vi "LVIS_VerifyTests.vi"(8 "Error In":errorcluster) -> (0 "Error Out":errorcluster)   [LabVIEW 2015]
doc: "Organizes the test and measurement data and verifies it is valid."
uses:
  Globals/LVIS_IsGlobal.vi
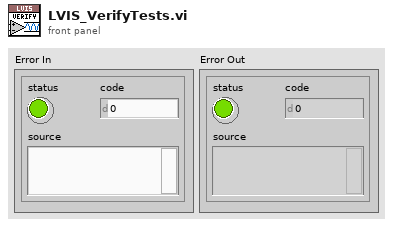
[diagram p1: front panel]
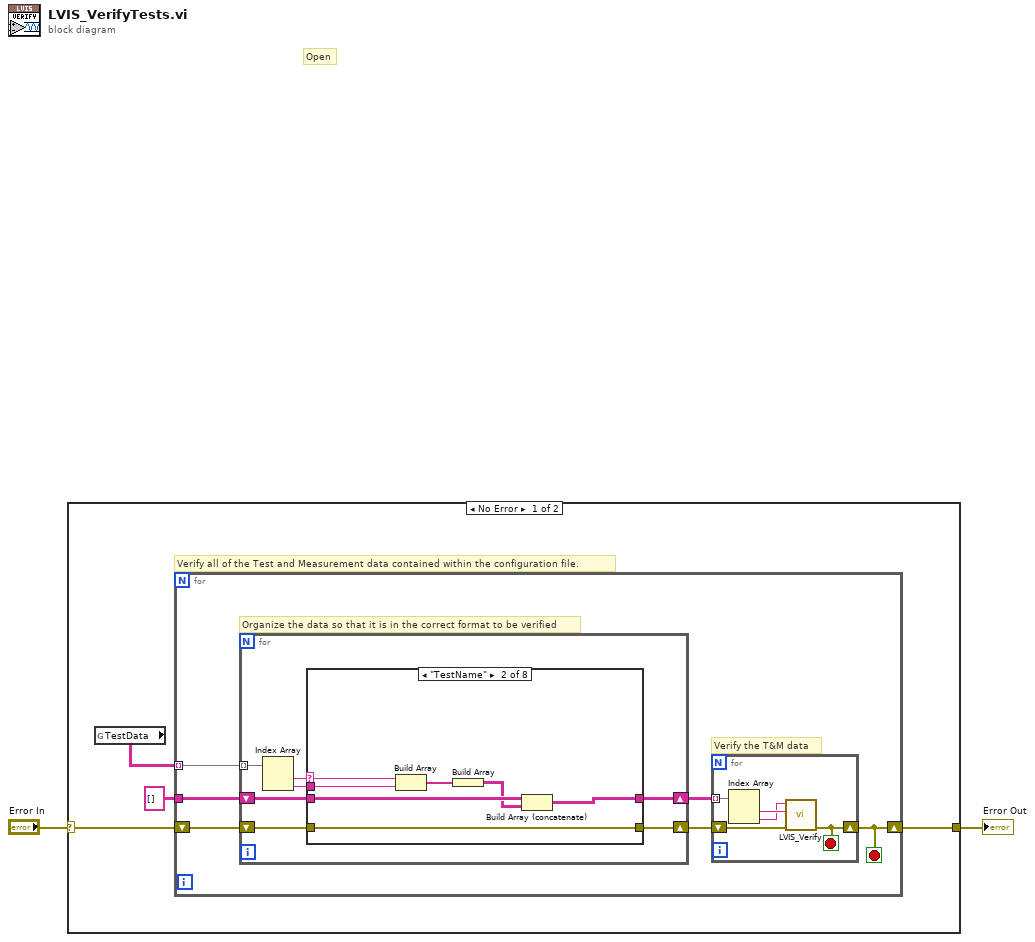
[diagram p0: block diagram]
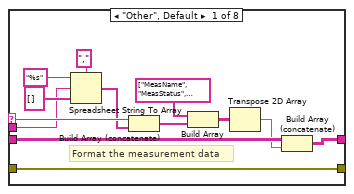
[diagram p2: hidden frame]
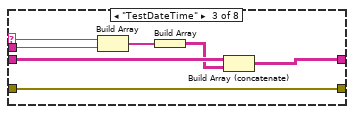
[diagram p3: hidden frame]
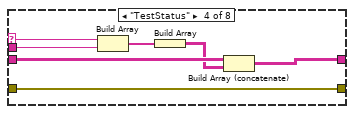
[diagram p4: hidden frame]
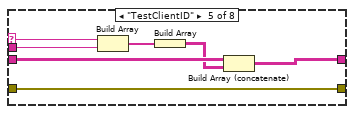
[diagram p5: hidden frame]
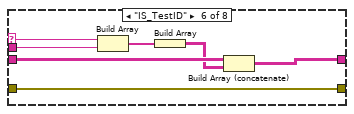
[diagram p6: hidden frame]
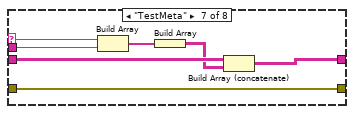
[diagram p7: hidden frame]
diagram:
  # "Open"
  n1 = case shown="No Error" "Error In" {
    selector: "Error In" -> [w3 w82]
    tunnel: [w5 w82] -> w2
    frame No Error {
      # "Verify all of the Test and Measurement data contained within the configuration file."
      n2 = global read "LVIS_IsGlobal.vi" "TestData"() -> (w6:string[][][])
      n3 = for {
        tunnel: w6 -> [w12] mode=indexing
        shift-right: [w8] -> w5
        shift-left: w3 -> [w10]
        tunnel: string[][] [] ("TestData") -> [w7]
        stop <- w8 stop-if-true
        # "Verify the T&M data"
        # "Organize the data so that it is in the correct format to be verified"
        n4 = for {
          tunnel: w12 -> [w24] mode=indexing
          shift-right: [w21] -> w11
          shift-left: w10 -> [w20]
          shift-right: [w18] -> w9
          shift-left: w7 -> [w19]
          n5 = Index Array(array=w24) -> (element #1=w23:string, element #2=w22:string)  [unwired: 2 in]
          n6 = case shown="\"TestName\"" w23 {
            selector: w23 -> [w36 w44 w51 w58 w65 w72 w79 _]
            tunnel: w22 -> [w29 w43 w50 w57 w64 w71 w78 _]
            tunnel: w20 -> [w32 w42 w49 w56 w63 w70 w77 w81]
            tunnel: [w32 w42 w49 w56 w63 w70 w77 w81] -> w21
            tunnel: w19 -> [w28 w40 w47 w54 w61 w68 w75 w80]
            tunnel: [w27 w38 w45 w52 w59 w66 w73 w80] -> w18
            frame "Other", Default {
              # "Format the measurement data"
              n7 = Spreadsheet String To Array(delimiter (Tab)=",", format string="%s" ("spreadsheet string"), spreadsheet string=w29, array type (2D Dbl)=string[] []) -> (array=w35:string[])
              n8 = Build Array (concatenate)(w36, w35) -> (w34:string[])
              n9 = Build Array(string[] ["MeasName", "MeasStatus", "MeasType", "LL", "LL Comp", "HL", "HL Comp", "Units", "MeasMeta"], w34) -> (w33:string[][])
              n10 = Transpose 2D Array(2D array=w33) -> (transposed array=w26:string[][])
              n11 = Build Array (concatenate)(w28, w26) -> (w27:string[][])
            }
            frame "TestName" {
              n12 = Build Array(w44, w43) -> (w41:string[])
              n13 = Build Array(w41) -> (w39:string[][])
              n14 = Build Array (concatenate)(w40, w39) -> (w38:string[][])
            }
            frame "TestDateTime" {
              n15 = Build Array(w51, w50) -> (w48:string[])
              n16 = Build Array(w48) -> (w46:string[][])
              n17 = Build Array (concatenate)(w47, w46) -> (w45:string[][])
            }
            frame "TestStatus" {
              n18 = Build Array(w58, w57) -> (w55:string[])
              n19 = Build Array(w55) -> (w53:string[][])
              n20 = Build Array (concatenate)(w54, w53) -> (w52:string[][])
            }
            frame "TestClientID" {
              n21 = Build Array(w65, w64) -> (w62:string[])
              n22 = Build Array(w62) -> (w60:string[][])
              n23 = Build Array (concatenate)(w61, w60) -> (w59:string[][])
            }
            frame "IS_TestID" {
              n24 = Build Array(w72, w71) -> (w69:string[])
              n25 = Build Array(w69) -> (w67:string[][])
              n26 = Build Array (concatenate)(w68, w67) -> (w66:string[][])
            }
            frame "TestMeta" {
              n27 = Build Array(w79, w78) -> (w76:string[])
              n28 = Build Array(w76) -> (w74:string[][])
              n29 = Build Array (concatenate)(w75, w74) -> (w73:string[][])
            }
            frame "" {
              # "Blank entry due to different 2D array sizes"
            }
          }
        }
        n30 = for {
          tunnel: w9 -> [w16] mode=indexing
          shift-right: [w13] -> w8
          shift-left: w11 -> [w17]
          stop <- w13 stop-if-true
          n31 = Index Array(array=w16) -> (element #1=w15:string, element #2=w14:string)  [unwired: 2 in]
          n32 = call "LVIS_Verify.vi"("Error In"=w17, "Field Name"=w15, "Field Value In"=w14) -> ("Error Out"=w13:errorcluster)  [unwired: 7 in, 1 out]
        }
      }
    }
    frame Error {
    }
  }
  "Error Out" <- w2
